vi "Serialize.vi"(7 "DestinationFolder":path, 8 "error in":errorcluster, 9 "OwningElement in":refnum<k20>, 10 "Document in":refnum<k20>, 11 "OperationRun in":refnum<class "OperationRun.lvclass">) -> (0 "error out":errorcluster, 1 "OwningElement out":refnum<k20>, 2 "Document out":refnum<k20>, 3 "OperationRun out":refnum<class "OperationRun.lvclass">)   [LabVIEW 2021, in "ProligentXMLGenerator.lvlib" / "OperationRun.lvclass"]
uses:
  OperationRun.lvclass
  OperationRun.lvclass/OperationRun.ctl
  <vilib>/xml/NI_XML.lvlib
  Base/DOMSupport/DOMSupport.lvlib
  Model/Characteristic/Characteristic.lvclass
  Model/CustomData/CustomData.lvclass
  Model/Document/Document.lvclass
  SequenceRun/SequenceRun/SequenceRun.lvclass
  Failure/FailureReference/FailureReference.lvclass
  SequenceRun/SequenceRunReference/SequenceRunReference.lvclass
  <vilib>/xml/Close Reference(Node).vi
  Base/ProcessFullName/ProcessFullName.lvclass
  C:/Projects/proligent-xml-generator-labview/src/ProligentXMLGenerator/Base/NonEmptyString/NonEmptyString.lvclass
  C:/Projects/proligent-xml-generator-labview/src/ProligentXMLGenerator/Base/String/String.lvclass
  C:/Projects/proligent-xml-generator-labview/src/ProligentXMLGenerator/Base/Attribute/Attribute.lvclass
  C:/Projects/proligent-xml-generator-labview/src/ProligentXMLGenerator/Base/ProcessFullName/ProcessFullName.lvclass
  Base/NonEmptyString_64/NonEmptyString_64.lvclass
  C:/Projects/proligent-xml-generator-labview/src/ProligentXMLGenerator/Base/NonEmptyString_64/NonEmptyString_64.lvclass
  Base/NonEmptyString_65/NonEmptyString_65.lvclass
  C:/Projects/proligent-xml-generator-labview/src/ProligentXMLGenerator/Base/NonEmptyString_65/NonEmptyString_65.lvclass
  Base/FullName/FullName.lvclass
  C:/Projects/proligent-xml-generator-labview/src/ProligentXMLGenerator/Base/FullName/FullName.lvclass
  Base/NonEmptyString_255/NonEmptyString_255.lvclass
  C:/Projects/proligent-xml-generator-labview/src/ProligentXMLGenerator/Base/NonEmptyString_255/NonEmptyString_255.lvclass
  Base/Guid/Guid.lvclass
  C:/Projects/proligent-xml-generator-labview/src/ProligentXMLGenerator/Base/Guid/Guid.lvclass
  Base/ExecutionStatus/ExecutionStatus.lvclass
  C:/Projects/proligent-xml-generator-labview/src/ProligentXMLGenerator/Base/ExecutionStatus/ExecutionStatus.lvclass
  Base/DateTime/DateTime.lvclass
  C:/Projects/proligent-xml-generator-labview/src/ProligentXMLGenerator/Base/DateTime/DateTime.lvclass
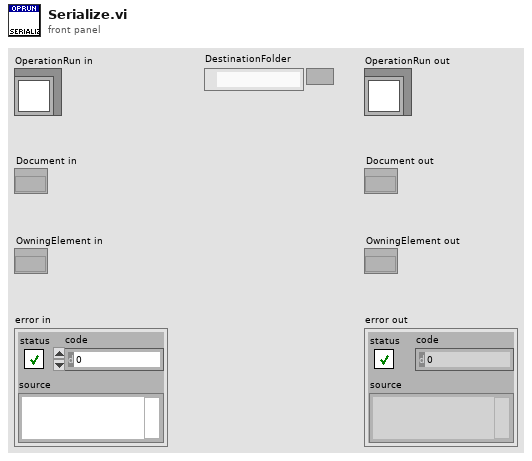
[diagram p1: front panel]
types:
  T1 = typedef "ProligentXMLGenerator.lvlib/OperationRun.lvclass/Data.ctl" = cluster{"Name":string, "Characteristics":refnum<class "Characteristic.lvclass">[], "Documents":refnum<class "Document.lvclass">[], "SequenceRuns":refnum<class "SequenceRun.lvclass">[], "FailureReferences":refnum<class "FailureReference.lvclass">[], "SequenceRunReferences":refnum<class "SequenceRunReference.lvclass">[], "CustomData":refnum<class "CustomData.lvclass">, "OperationRunId":refnum<class "Guid.lvclass">, "ProcessFullName":refnum<class "ProcessFullName.lvclass">, "ProcessVersion":refnum<class "NonEmptyString_64.lvclass">, "OperationName":refnum<class "NonEmptyString_65.lvclass">, "StationFullName":refnum<class "FullName.lvclass">, "User":refnum<class "NonEmptyString_255.lvclass">, "CallingOperationRunId":refnum<class "Guid.lvclass">, "OperationStatus":refnum<class "ExecutionStatus.lvclass">, "OperationRunStartTime":refnum<class "DateTime.lvclass">, "OperationRunEndTime":refnum<class "DateTime.lvclass">, "TimeZoneInfoId":string}
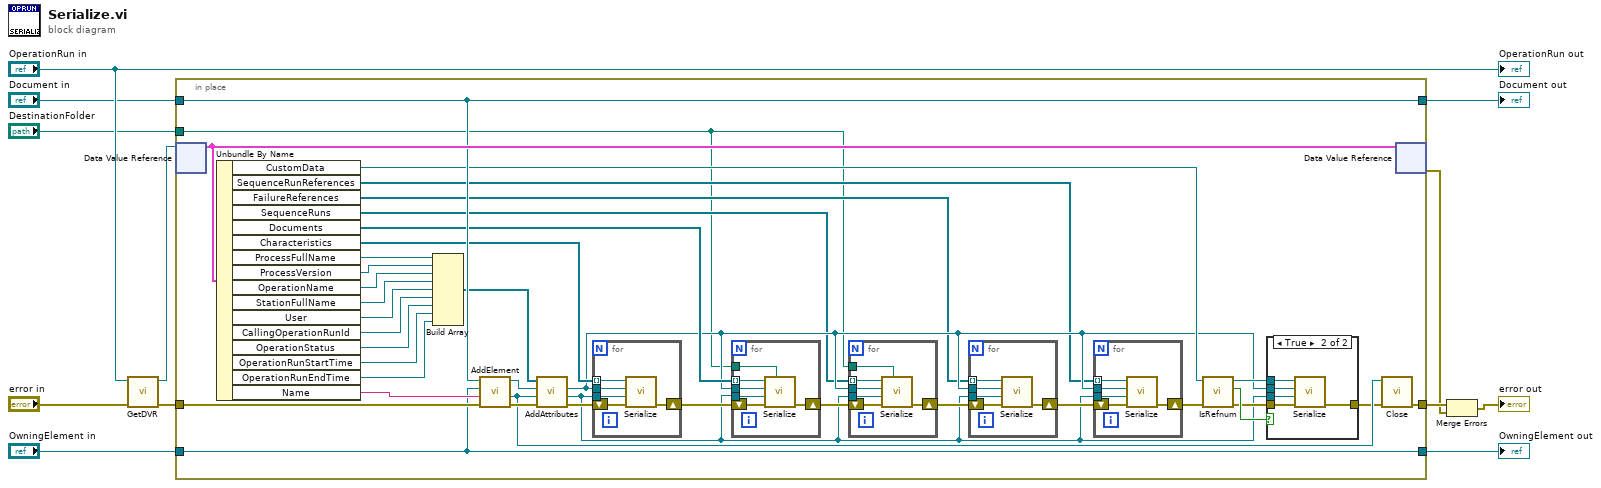
[diagram p0: block diagram]
diagram:
  n1 = call "GetDVR.vi"("error in"="error in", "OperationRun"="OperationRun in") -> ("error out"=w4:errorcluster, "DVRReference"=w3:refnum<data-value>)  [unwired: 8 in]
  n2 = in-place "In Place Element Structure" {
    in-place-border: [w50] -> w5
    in-place-border: "Document in" -> [w45]
    in-place-border: w4 -> [w49]
    in-place-border: "OwningElement in" -> [w47]
    in-place-border: [w47] -> w7
    in-place-border: [w45] -> w6
    in-place-border: "DestinationFolder" -> [w13]
    n3 = in-place-dvr #1(w3) -> (w46:T1)  [unwired: 1 out]
    n4 = Unbundle By Name(w46) -> ("CustomData"=w24:refnum<class "CustomData.lvclass">, "SequenceRunReferences"=w17:refnum<class "SequenceRunReference.lvclass">[], "FailureReferences"=w18:refnum<class "FailureReference.lvclass">[], "SequenceRuns"=w19:refnum<class "SequenceRun.lvclass">[], "Documents"=w23:refnum<class "Document.lvclass">[], "Characteristics"=w34:refnum<class "Characteristic.lvclass">[], "ProcessFullName"=w43:refnum<class "ProcessFullName.lvclass">, "ProcessVersion"=w16:refnum<class "NonEmptyString_64.lvclass">, "OperationName"=w42:refnum<class "NonEmptyString_65.lvclass">, "StationFullName"=w15:refnum<class "FullName.lvclass">, "User"=w41:refnum<class "NonEmptyString_255.lvclass">, "CallingOperationRunId"=w14:refnum<class "Guid.lvclass">, "OperationStatus"=w40:refnum<class "ExecutionStatus.lvclass">, "OperationRunStartTime"=w39:refnum<class "DateTime.lvclass">, "OperationRunEndTime"=w33:refnum<class "DateTime.lvclass">, "Name"=w48:string)
    n5 = Build Array(w43, w16, w42, w15, w41, w14, w40, w39, w33) -> (w36:refnum<class "Attribute.lvclass">[])
    n6 = call "AddElement.vi"("error in"=w49, "Name"=w48, "OwningElement in"=w47, "Document in"=w45) -> ("error out"=w44:errorcluster, "NewElement"=w38:refnum<k20>, "Document out"=w37:refnum<k20>)  [unwired: 4 in, 1 out]
    n7 = call "AddAttributes.vi"("error in"=w44, "OwningElement in"=w38, "Document in"=w37, "Attributes"=w36) -> ("error out"=w35:errorcluster, "OwningElement out"=w21:refnum<k20>, "Document out"=w22:refnum<k20>)  [unwired: 5 in]
    n8 = for {
      tunnel: w34 -> [w83] mode=indexing
      tunnel: w21 -> [w81]
      tunnel: w22 -> [w82]
      shift-right: [w79] -> w31
      shift-left: w35 -> [w80]
      n9 = call "Serialize.vi"("error in"=w80, "OwningElement in"=w81, "Document in"=w82, "DocumentType in"=w83) -> ("error out"=w79:errorcluster)  [unwired: 4 in, 3 out]
    }
    n10 = for {
      tunnel: w23 -> [w78] mode=indexing
      tunnel: w21 -> [w76]
      tunnel: w22 -> [w77]
      shift-right: [w74] -> w32
      shift-left: w31 -> [w75]
      tunnel: w13 -> [w73]
      n11 = call "Serialize.vi"("DestinationFolder"=w73, "error in"=w75, "OwningElement in"=w76, "Document in"=w77, "DocumentType in"=w78) -> ("error out"=w74:errorcluster)  [unwired: 3 in, 3 out]
    }
    n12 = for {
      tunnel: w19 -> [w72] mode=indexing
      tunnel: w21 -> [w70]
      tunnel: w22 -> [w71]
      shift-right: [w68] -> w30
      shift-left: w32 -> [w69]
      tunnel: w13 -> [w67]
      n13 = call "Serialize.vi"("DestinationFolder"=w67, "error in"=w69, "OwningElement in"=w70, "Document in"=w71, "SequenceRun in"=w72) -> ("error out"=w68:errorcluster)  [unwired: 3 in, 3 out]
    }
    n14 = for {
      tunnel: w18 -> [w66] mode=indexing
      tunnel: w21 -> [w64]
      tunnel: w22 -> [w65]
      shift-right: [w62] -> w29
      shift-left: w30 -> [w63]
      n15 = call "Serialize.vi"("error in"=w63, "OwningElement in"=w64, "Document in"=w65, "FailureReference in"=w66) -> ("error out"=w62:errorcluster)  [unwired: 4 in, 3 out]
    }
    n16 = for {
      tunnel: w17 -> [w61] mode=indexing
      tunnel: w21 -> [w59]
      tunnel: w22 -> [w60]
      shift-right: [w57] -> w28
      shift-left: w29 -> [w58]
      n17 = call "Serialize.vi"("error in"=w58, "OwningElement in"=w59, "Document in"=w60, "SequenceRunReference in"=w61) -> ("error out"=w57:errorcluster)  [unwired: 4 in, 3 out]
    }
    n18 = call "IsRefnum.vi"("error in"=w28, "CustomDataType in"=w24) -> ("error out"=w26:errorcluster, "IsRefnum"=w27:bool, "CustomDataType out"=w25:refnum<class "CustomData.lvclass">)  [unwired: 7 in]
    n19 = case shown="True" w27 {
      tunnel: w26 -> [w51 w56]
      tunnel: [w51 w55] -> w20
      tunnel: w25 -> [_ w54]
      tunnel: w22 -> [_ w53]
      tunnel: w21 -> [_ w52]
      frame False {
      }
      frame True {
        n20 = call "Serialize.vi"("error in"=w56, "OwningElement in"=w52, "Document in"=w53, "CustomDataType in"=w54) -> ("error out"=w55:errorcluster)  [unwired: 4 in, 3 out]
      }
    }
    n21 = call-poly <vilib>:"Close.vi"("error in (no error)"=w20, "node"=w38) -> ("error out"=w50:errorcluster)  [unwired: 7 in]
    n22 = in-place-dvr #1(w46) -> (w2:errorcluster)  [unwired: 1 out]
  }
  "Document out" <- w6
  "OwningElement out" <- w7
  n23 = Merge Errors(w5, w2) -> (→"error out":errorcluster)
  "OperationRun out" <- "OperationRun in"
